vi "Get Alarming Enqueuer.vi"(11 "Action Point in":refnum<class "Action Point.lvclass">) -> (2 "Alarming Enqueuer":refnum<class "Message Enqueuer.lvclass">, 3 "Action Point out":refnum<class "Action Point.lvclass">)   [LabVIEW 2025, in "Action Point.lvclass"]
uses:
  Action Point.lvclass
  <vilib>/ActorFramework/Message Enqueuer/Message Enqueuer.lvclass
  Action Point.lvclass/Action Point.ctl
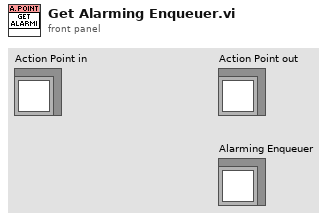
[diagram p1: front panel]
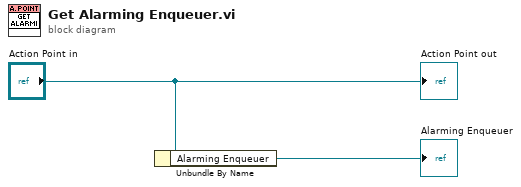
[diagram p0: block diagram]
diagram:
  n1 = Unbundle By Name("Action Point in") -> ("Alarming Enqueuer"=→"Alarming Enqueuer":refnum<class "Message Enqueuer.lvclass">)
  "Action Point out" <- "Action Point in"
